vi "Add_Target.vi"(11 "Error_In":errorcluster) -> (4 "Target_Specification_Out":T1={"Target_Name"="LM233", "Register_Name"=["Register A", "Register B"], "Register_Address"=[0.0, 1.0], "Vmin"=0.0, "Vmax"=5.0, "Off_Set (uS)"=10.0, "T_HD_STA (uS)"=5.0, "T_HD_DAT (uS)"=5.0, "T_SU_DAT (uS)"=0.25, "Frequency (kHz)"=100.0, "T_SU_STO"=4.0, "T_Off (uS)"=5.0, "T_On (uS)"=5.0, "T_BUF"=5.0, "Sample_Per_Us"=1000.0, "Target_Type"=0, "Target_Address"=21} {"Target_Address" format="%x"; "Target_Type" items=["10 Bit Address", "7 Bit Address"]}, 15 "Error_Out":errorcluster)   [LabVIEW 2023]
uses:
  Controls/Add_Target_Specification_.ctl
  Controls/Menu_Ring.ctl
  Controls/Button.ctl
  Controls/Queue_Operation.ctl
  Controls/State_and_Data.ctl
  Drivers/Queue_Driver/QD_Main.vi
panel:
  in  "Add":T3
  in  "Target_Specification_In":T1 {"Target_Address" format="%x"; "Target_Type" items=["10 Bit Address", "7 Bit Address"]}
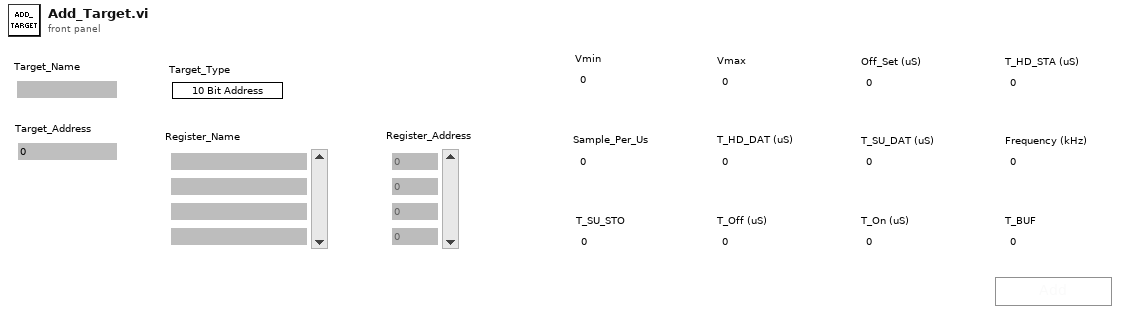
[diagram p1: front panel]
types:
  T1 = typedef "Add_Target_Specification_.ctl" = cluster{"Target_Name":string, "Register_Name":string[], "Register_Address":dbl[], "Vmin":dbl, "Vmax":dbl, "Off_Set (uS)":dbl, "T_HD_STA (uS)":dbl, "T_HD_DAT (uS)":dbl, "T_SU_DAT (uS)":dbl, "Frequency (kHz)":dbl, "T_SU_STO":dbl, "T_Off (uS)":dbl, "T_On (uS)":dbl, "T_BUF":dbl, "Sample_Per_Us":dbl, "Target_Type":T2, "Target_Address":u16}
  T2 = typedef "Menu_Ring.ctl" = u16
  T3 = typedef "Button.ctl" = bool
  T4 = typedef "Queue_Operation.ctl" = enum16{"Obtain_Queue", "Enqueue", "Enqueue_First", "Enqueue_N", "Lossy_Enqueue", "Preview", "Queue_Status", "Dequeue", "Flush", "Release_Queue"}
  T5 = typedef "State_and_Data.ctl" = cluster{"State":string, "Data":variant}
  T6 = enum32{"Invalid", "Standard", "Closed", "Hidden", "Minimized", "Maximized"}
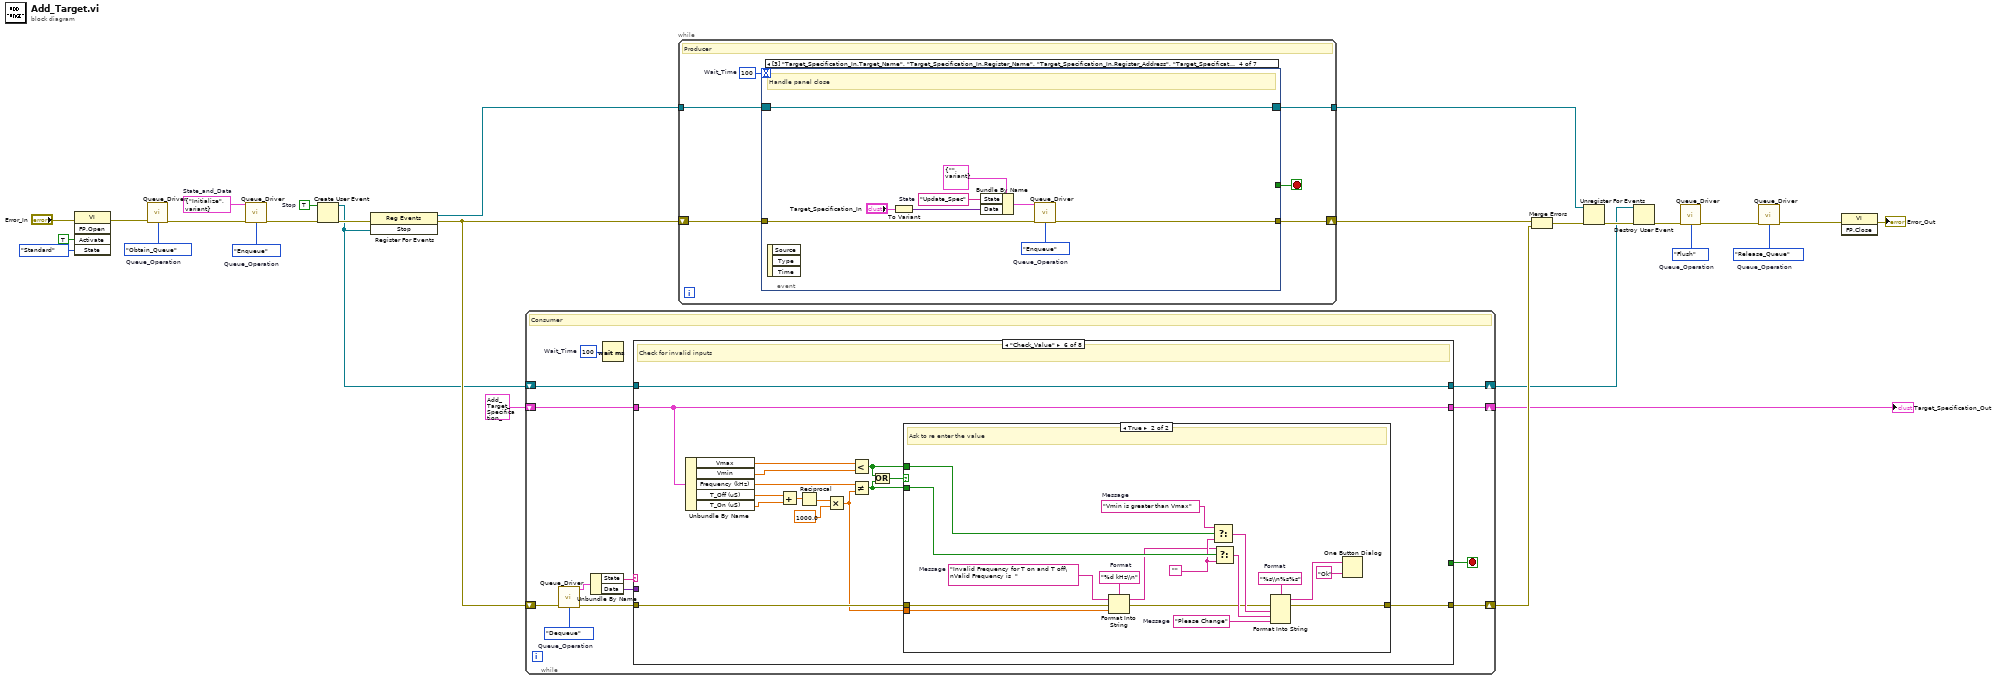
[diagram p0: block diagram]
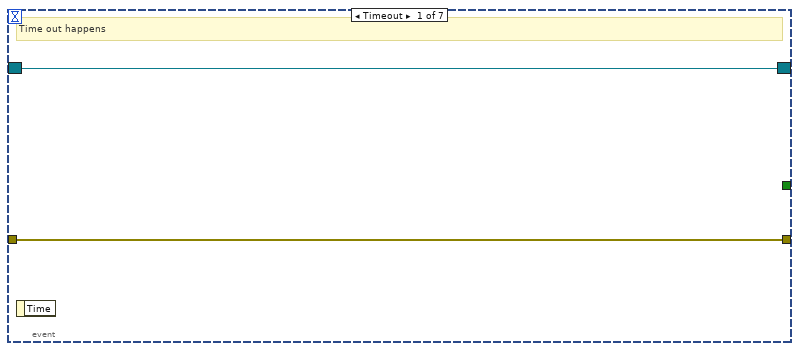
[diagram p2: hidden frame]
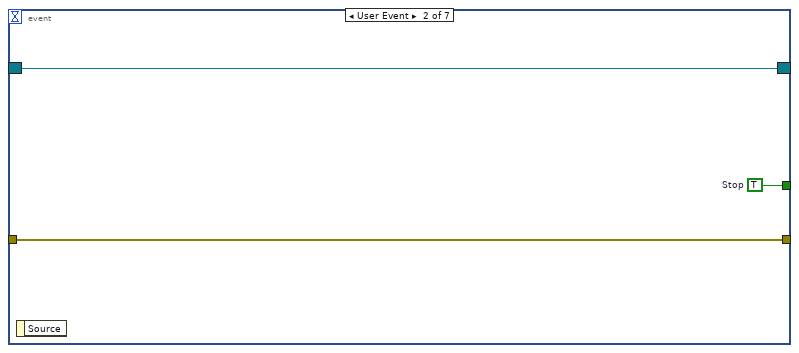
[diagram p3: hidden frame]
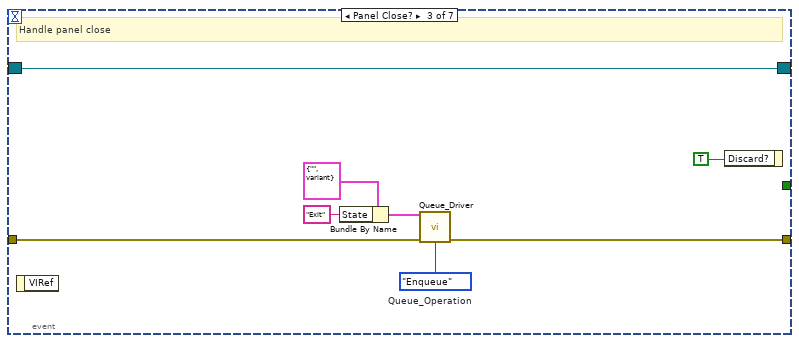
[diagram p4: hidden frame]
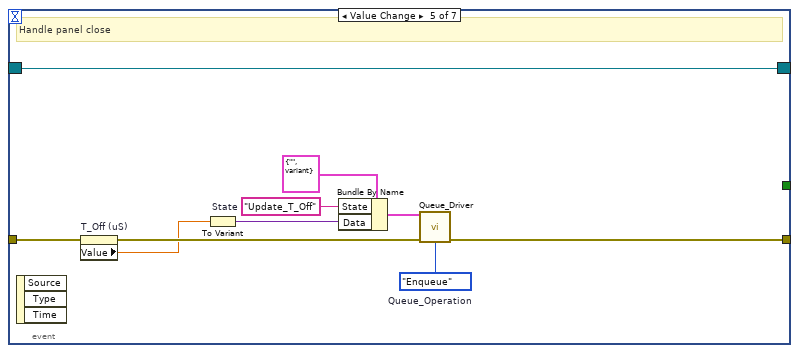
[diagram p5: hidden frame]
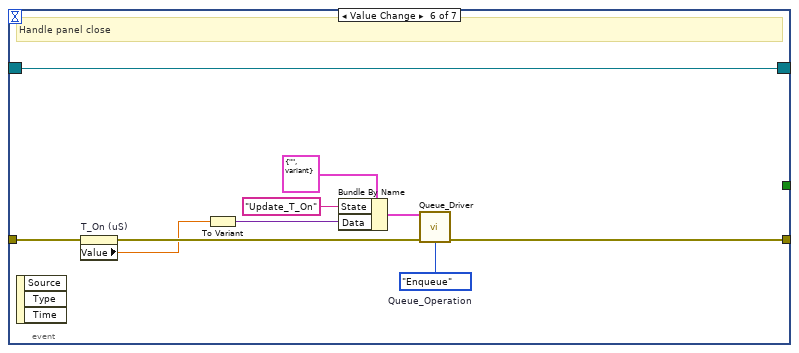
[diagram p6: hidden frame]
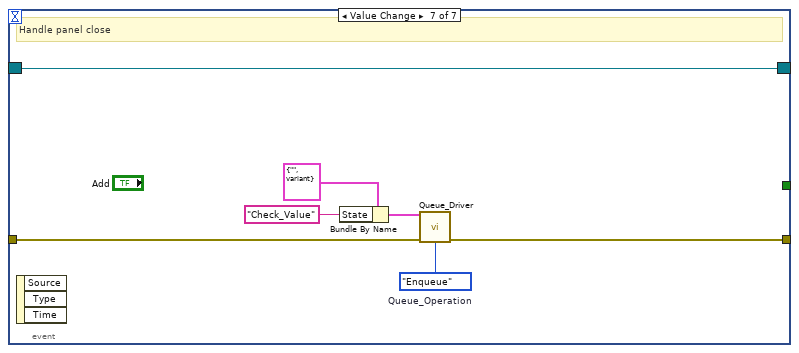
[diagram p7: hidden frame]
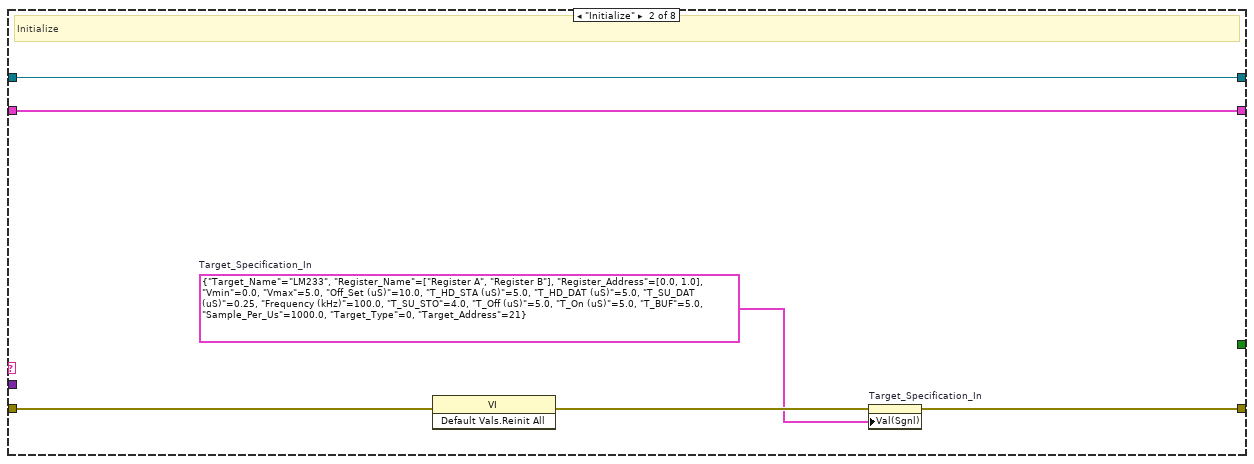
[diagram p9: hidden frame]
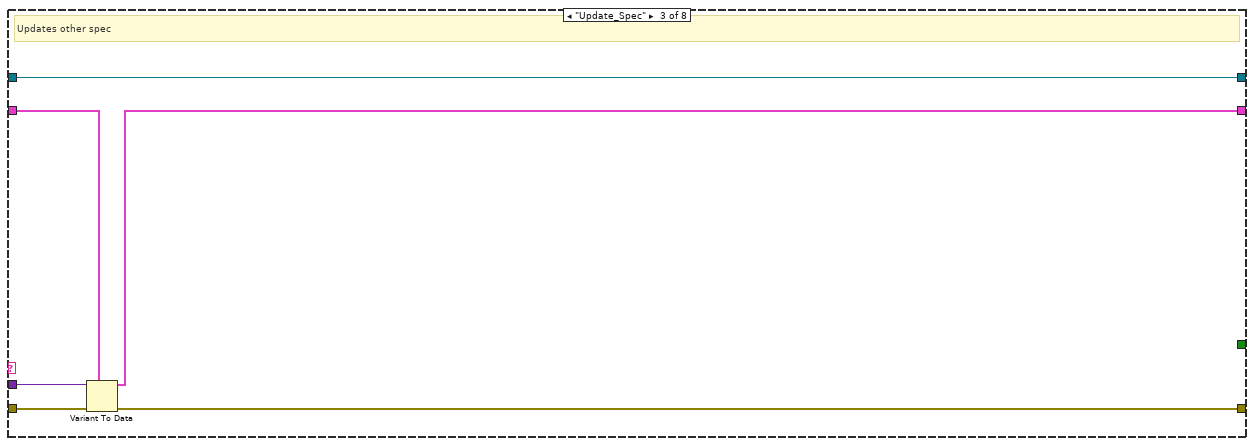
[diagram p10: hidden frame]
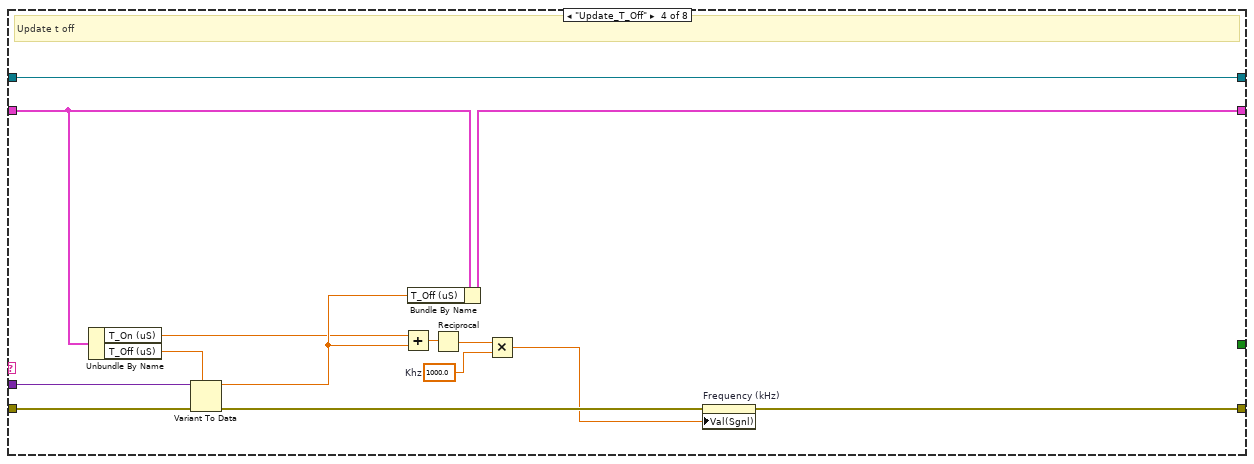
[diagram p11: hidden frame]
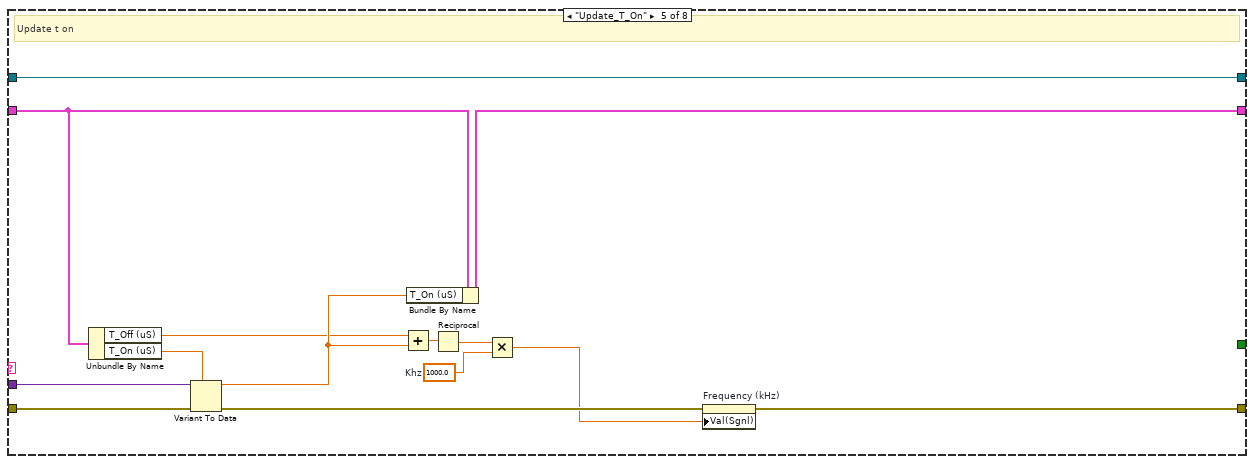
[diagram p12: hidden frame]
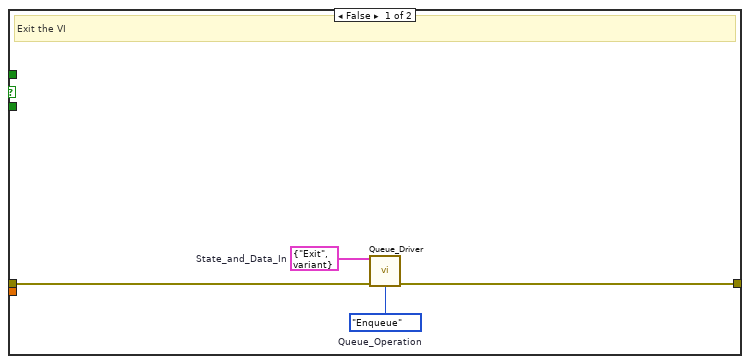
[diagram p13: hidden frame]
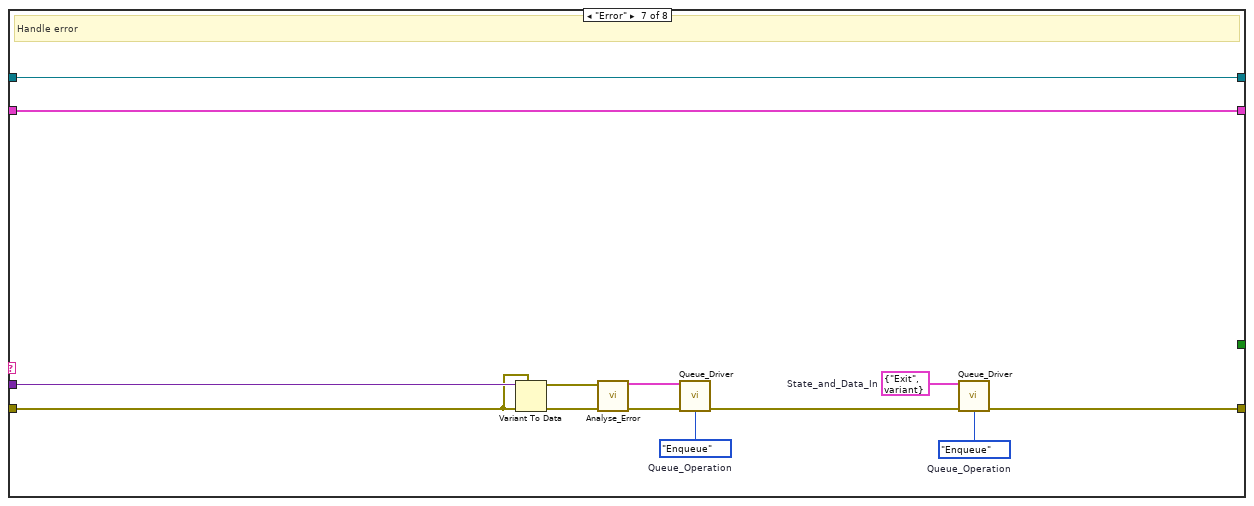
[diagram p14: hidden frame]
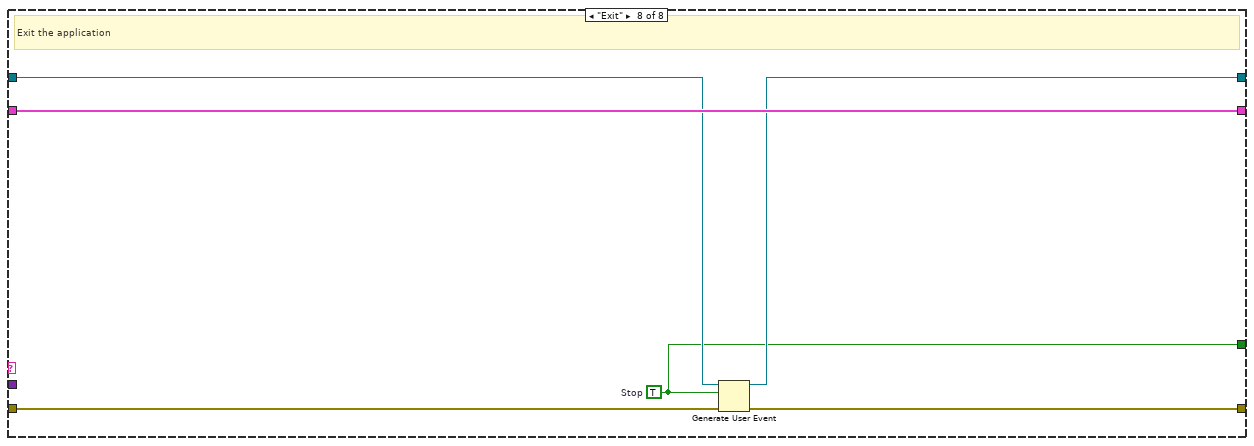
[diagram p15: hidden frame]
diagram:
  w8 = Queue_Operation."Release_Queue"  # Queue_Operation
  w9 = Queue_Operation."Flush"  # Queue_Operation
  w19 = TRUE  # Stop
  w21 = T5 {"State"="Initialize", "Data"=variant}  # State_and_Data
  w22 = Queue_Operation."Enqueue"  # Queue_Operation
  w23 = Queue_Operation."Obtain_Queue"  # Queue_Operation
  n1 = invoke class="VI" method="FP.Open"(error in="Error_In", "Activate"=TRUE ("Activate?"), "State"=T6."Standard") -> (error out=w4:errorcluster)  [unwired: 2 in, 4 out]
  n2 = call-poly "Queue_Driver.vi"("Error_In"=w4, "Queue_Operation"=w23) -> ("Error_Out"=w24:errorcluster)  [unwired: 11 in, 2 out]
  n3 = call-poly "Queue_Driver.vi"("State_and_Data_In"=w21, "Error_In"=w24, "Queue_Operation"=w22) -> ("Error_Out"=w7:errorcluster)  [unwired: 10 in, 2 out]
  n4 = Create User Event(user event datatype=w19, error in=w7) -> (user event=w5:refnum<user-event>, error out=w20:errorcluster)
  n5 = register-events(error in=w20, w5) -> (reference out=w18:refnum<event-registration>, error out=w6:errorcluster)  [unwired: 1 in]
  n6 = while {
    shift-right: [w33] -> w12
    shift-left: w5 -> [w34]
    shift-right: [w32] -> w1
    shift-left: T1 {"Target_Name"="LM233", "Register_Name"=["Register A", "Register B"], "Register_Address"=[0.0, 1.0], "Vmin"=0.0, "Vmax"=5.0, "Off_Set (uS)"=10.0, "T_HD_STA (uS)"=5.0, "T_HD_DAT (uS)"=5.0, "T_SU_DAT (uS)"=0.25, "Frequency (kHz)"=100.0, "T_SU_STO"=4.0, "T_Off (uS)"=5.0, "T_On (uS)"=5.0, "T_BUF"=5.0, "Sample_Per_Us"=1000.0, "Target_Type"=0, "Target_Address"=21} ("Target_Specification_In") -> [w35]
    shift-right: [w31] -> w16
    shift-left: w6 -> [w41]
    stop <- w30 stop-if-true
    w29 = u32 100  # Wait_Time
    w39 = Queue_Operation."Dequeue"  # Queue_Operation
    # "Consumer"
    n7 = call-poly "Queue_Driver.vi"("Error_In"=w41, "Queue_Operation"=w39) -> ("State_and_Data_Out"=w38:T5, "Error_Out"=w40:errorcluster)  [unwired: 11 in, 1 out]
    n8 = Unbundle By Name(w38) -> ("State"=w37:string, "Data"=w36:variant)
    n9 = Wait (ms)(milliseconds to wait=w29) -> ()  [unwired: 1 out]
    n10 = case shown="\"Check_Value\"" w37 {
      tunnel: [w44 w46 w54 w58 w72 w89 w124 w138] -> w31
      tunnel: w40 -> [w44 w49 w56 w70 w84 w100 w132 w140]
      tunnel: w36 -> [_ _ w53 w67 w81 _ w133 _]
      tunnel: w35 -> [w43 w48 w52 w66 w80 w98 w129 w139]
      tunnel: [w43 w48 w51 w64 w78 w98 w129 w139] -> w32
      tunnel: w34 -> [w42 w50 w55 w69 w83 w99 w134 w137]
      tunnel: [w42 w50 w55 w69 w83 w99 w134 w136] -> w33
      tunnel: [_ _ _ _ _ _ _ w135] -> w30
      frame Default {
      }
      frame "Initialize" {
        w45 = T1 {"Target_Name"="LM233", "Register_Name"=["Register A", "Register B"], "Register_Address"=[0.0, 1.0], "Vmin"=0.0, "Vmax"=5.0, "Off_Set (uS)"=10.0, "T_HD_STA (uS)"=5.0, "T_HD_DAT (uS)"=5.0, "T_SU_DAT (uS)"=0.25, "Frequency (kHz)"=100.0, "T_SU_STO"=4.0, "T_Off (uS)"=5.0, "T_On (uS)"=5.0, "T_BUF"=5.0, "Sample_Per_Us"=1000.0, "Target_Type"=0, "Target_Address"=21}  # Target_Specification_In
        # "Initialize"
        n11 = invoke class="VI" method="Default Vals.Reinit All"(error in=w49) -> (error out=w47:errorcluster)  [unwired: 2 in, 2 out]
        n12 = property on="Target_Specification_In" class="Clust (strict)"(error in=w47, "Val(Sgnl)"=w45) -> (error out=w46:errorcluster)  [unwired: 1 in, 1 out]
      }
      frame "Update_Spec" {
        # "Updates other spec"
        n13 = Variant To Data(error in=w56, type=w52, Variant=w53) -> (data=w51:T1, error out=w54:errorcluster)
      }
      frame "Update_T_Off" {
        w61 = 1000.0  # Khz
        # "Update t off"
        n14 = Unbundle By Name(w66) -> ("T_On (uS)"=w59:dbl, "T_Off (uS)"=w65:dbl)
        n15 = Variant To Data(error in=w70, type=w65, Variant=w67) -> (data=w60:dbl, error out=w68:errorcluster)
        n16 = Add(x=w59, y=w60) -> (x+y=w63:dbl)
        n17 = Bundle By Name(cluster=w66, "T_Off (uS)"=w60) -> (w64:T1)
        n18 = Reciprocal(x=w63) -> (1/x=w62:dbl)
        n19 = Multiply(x=w62, y=w61) -> (x*y=w57:dbl)
        n20 = property on="Frequency (kHz)" class="DigNum (strict)"(error in=w68, "Val(Sgnl)"=w57) -> (error out=w58:errorcluster)  [unwired: 1 in, 1 out]
      }
      frame "Update_T_On" {
        w75 = 1000.0  # Khz
        # "Update t on"
        n21 = Unbundle By Name(w80) -> ("T_Off (uS)"=w73:dbl, "T_On (uS)"=w79:dbl)
        n22 = Variant To Data(error in=w84, type=w79, Variant=w81) -> (data=w74:dbl, error out=w82:errorcluster)
        n23 = Add(x=w73, y=w74) -> (x+y=w77:dbl)
        n24 = Bundle By Name(cluster=w80, "T_On (uS)"=w74) -> (w78:T1)
        n25 = Reciprocal(x=w77) -> (1/x=w76:dbl)
        n26 = Multiply(x=w76, y=w75) -> (x*y=w71:dbl)
        n27 = property on="Frequency (kHz)" class="DigNum (strict)"(error in=w82, "Val(Sgnl)"=w71) -> (error out=w72:errorcluster)  [unwired: 1 in, 1 out]
      }
      frame "Check_Value" {
        # "Check for invalid inputs"
        n28 = Unbundle By Name(w98) -> ("Vmax"=w97:dbl, "Vmin"=w96:dbl, "Frequency (kHz)"=w90:dbl, "T_Off (uS)"=w95:dbl, "T_On (uS)"=w94:dbl)
        n29 = Add(x=w95, y=w94) -> (x+y=w93:dbl)
        n30 = Reciprocal(x=w93) -> (1/x=w92:dbl)
        n31 = Multiply(x=w92, y=1000.0) -> (x*y=w88:dbl)
        n32 = Less?(x=w97, y=w96) -> (x < y?=w86:bool)
        n33 = Not Equal?(x=w90, y=w88) -> (x != y?=w87:bool)
        n34 = Or(x=w86, y=w87) -> (x .or. y?=w85:bool)
        n35 = case shown="True" w85 {
          tunnel: w100 -> [w104 w121]
          tunnel: [w103 w120] -> w89
          tunnel: w86 -> [_ w117]
          tunnel: w87 -> [_ w114]
          tunnel: w88 -> [_ w108]
          frame False {
            w101 = T5 {"State"="Exit", "Data"=variant}  # State_and_Data_In
            w102 = Queue_Operation."Enqueue"  # Queue_Operation
            # "Exit the VI"
            n36 = call-poly "Queue_Driver.vi"("State_and_Data_In"=w101, "Error_In"=w104, "Queue_Operation"=w102) -> ("Error_Out"=w103:errorcluster)  [unwired: 10 in, 2 out]
          }
          frame True {
            w105 = "%s\\n%s%s"  # Format
            w106 = "%d kHz\\n"  # Format
            w111 = "Please Change"  # Message
            w112 = ""
            w109 = "Invalid Frequency for T on and T off\nValid Frequency is  "  # Message
            w116 = "Vmin is greater than Vmax"  # Message
            # "Ask to re enter the value"
            n37 = Format Into String(format string=w106, initial string=w109, error in=w121, w108) -> (resulting string=w107:string, error out=w110:errorcluster)
            n38 = Select(t=w116, s=w117, f=w112) -> (s? t:f=w115:string)
            n39 = Select(t=w107, s=w114, f=w112) -> (s? t:f=w113:string)
            n40 = Format Into String(format string=w105, error in=w110, w115, w113, w111) -> (resulting string=w119:string, error out=w120:errorcluster)  [unwired: 1 in]
            n41 = One Button Dialog(message=w119, button name ("OK")="Ok") -> ()  [unwired: 1 out]
          }
        }
      }
      frame "Error" {
        w122 = T5 {"State"="Exit", "Data"=variant}  # State_and_Data_In
        w123 = Queue_Operation."Enqueue"  # Queue_Operation
        w127 = Queue_Operation."Enqueue"  # Queue_Operation
        # "Handle error"
        n42 = Variant To Data(error in=w132, type=w132, Variant=w133) -> (data=w126:errorcluster, error out=w131:errorcluster)
        n43 = call "Analyse_Error.vi"("Erroe_Under_Analyse"=w126, "Error_In"=w131) -> ("State_and_Data"=w125:T5, "Error_Out"=w130:errorcluster)  [unwired: 12 in]
        n44 = call-poly "Queue_Driver.vi"("State_and_Data_In"=w125, "Error_In"=w130, "Queue_Operation"=w127) -> ("Error_Out"=w128:errorcluster)  [unwired: 10 in, 2 out]
        n45 = call-poly "Queue_Driver.vi"("State_and_Data_In"=w122, "Error_In"=w128, "Queue_Operation"=w123) -> ("Error_Out"=w124:errorcluster)  [unwired: 10 in, 2 out]
      }
      frame "Exit" {
        w135 = TRUE  # Stop
        # "Exit the application"
        n46 = Generate User Event(user event=w137, event data cluster=w135, error in=w140) -> (user event out=w136:refnum<user-event>, error out=w138:errorcluster)  [unwired: 1 in]
      }
    }
  }
  "Target_Specification_Out" <- w1
  n47 = while {
    tunnel: w18 -> [w145]
    shift-right: [w144] -> w17
    shift-left: w6 -> [w146]
    tunnel: [w142] -> w14
    stop <- w141 stop-if-true
    w143 = 100  # Wait_Time
    # "Producer"
    n48 = event shown="[3] \"Target_Specification_In.Target_Name\", \"Target_Specification_In.Register_Name\", \"Target_Specification_In.Register_Address\", \"Target_Specification_In.Vmin\", \"Target_Specification_In.Vmax\", \"Target_Specification_In.T_HD_STA (uS)\", \"Target_Specification_In.T_SU_DAT (uS)\", \"Target_Specification_In.Frequency (kHz)\", \"Target_Specification_In.T_SU_STO\", \"Target_Specification_In.T_BUF\", \"Target_Specification_In.Sample_Per_Us\", \"Target_Specification_In.Target_Type\", \"Target_Specification_In.Target_Address\": Value Change" {
      selector: w145 -> [w147 w149 w152 w163 w173 w183 w190]
      dyn-events: [w147 w149 w152 w163 w173 w183 w190] -> w142
      timeout: w143 -> [_ _ _ _ _ _ _]
      tunnel: w146 -> [w148 w150 w156 w167 w177 w187 w194]
      tunnel: [w148 w150 w155 w166 w176 w186 w193] -> w144
      tunnel: [_ w151 _ _ _ _ _] -> w141
      event Timeout {
        # "Time out happens"
        n49 = event-data() -> ()  [unwired: 1 in, 1 out]
      }
      event User Event {
        w151 = TRUE  # Stop
        n50 = event-data() -> ()  [unwired: 1 in, 1 out]
      }
      event Panel Close? {
        w157 = Queue_Operation."Enqueue"  # Queue_Operation
        # "Handle panel close"
        n51 = event-data() -> ()  [unwired: 1 in, 1 out]
        n52 = Bundle By Name(cluster=T5 {"State"="", "Data"=variant} ("State_and_Data"), "State"="Exit") -> (w154:T5)
        n53 = call-poly "Queue_Driver.vi"("State_and_Data_In"=w154, "Error_In"=w156, "Queue_Operation"=w157) -> ("Error_Out"=w155:errorcluster)  [unwired: 10 in, 2 out]
        n54 = event-data("Discard?"=TRUE) -> ()  [unwired: 1 in, 1 out]
      }
      event Value Change {
        w162 = "Update_Spec"  # State
        w168 = Queue_Operation."Enqueue"  # Queue_Operation
        # "Handle panel close"
        n55 = event-data() -> ()  [unwired: 1 in, 3 out]
        n56 = To Variant(anything="Target_Specification_In") -> (Variant=w160:variant)
        n57 = Bundle By Name(cluster=T5 {"State"="", "Data"=variant} ("State_and_Data"), "State"=w162, "Data"=w160) -> (w165:T5)
        n58 = call-poly "Queue_Driver.vi"("State_and_Data_In"=w165, "Error_In"=w167, "Queue_Operation"=w168) -> ("Error_Out"=w166:errorcluster)  [unwired: 10 in, 2 out]
      }
      event Value Change {
        w172 = "Update_T_Off"  # State
        w178 = Queue_Operation."Enqueue"  # Queue_Operation
        # "Handle panel close"
        n59 = event-data() -> ()  [unwired: 1 in, 3 out]
        n60 = property on="T_Off (uS)" class="DigNum (strict)"(error in=w177) -> (error out=w170:errorcluster, "Value"=w169:dbl)  [unwired: 1 in, 1 out]
        n61 = To Variant(anything=w169) -> (Variant=w171:variant)
        n62 = Bundle By Name(cluster=T5 {"State"="", "Data"=variant} ("State_and_Data"), "State"=w172, "Data"=w171) -> (w175:T5)
        n63 = call-poly "Queue_Driver.vi"("State_and_Data_In"=w175, "Error_In"=w170, "Queue_Operation"=w178) -> ("Error_Out"=w176:errorcluster)  [unwired: 10 in, 2 out]
      }
      event Value Change {
        w188 = Queue_Operation."Enqueue"  # Queue_Operation
        # "Handle panel close"
        n64 = event-data() -> ()  [unwired: 1 in, 3 out]
        n65 = property on="T_On (uS)" class="DigNum (strict)"(error in=w187) -> (error out=w180:errorcluster, "Value"=w179:dbl)  [unwired: 1 in, 1 out]
        n66 = To Variant(anything=w179) -> (Variant=w181:variant)
        n67 = Bundle By Name(cluster=T5 {"State"="", "Data"=variant} ("State_and_Data"), "State"="Update_T_On", "Data"=w181) -> (w185:T5)
        n68 = call-poly "Queue_Driver.vi"("State_and_Data_In"=w185, "Error_In"=w180, "Queue_Operation"=w188) -> ("Error_Out"=w186:errorcluster)  [unwired: 10 in, 2 out]
      }
      event Value Change {
        w195 = Queue_Operation."Enqueue"  # Queue_Operation
        # "Handle panel close"
        n69 = event-data() -> ()  [unwired: 1 in, 3 out]
        n70 = Bundle By Name(cluster=T5 {"State"="", "Data"=variant} ("State_and_Data"), "State"="Check_Value") -> (w192:T5)
        n71 = call-poly "Queue_Driver.vi"("State_and_Data_In"=w192, "Error_In"=w194, "Queue_Operation"=w195) -> ("Error_Out"=w193:errorcluster)  [unwired: 10 in, 2 out]
      }
    }
  }
  n72 = Merge Errors(w17, w16) -> (w15:errorcluster)
  n73 = Unregister For Events(event registration refnum=w14, error in=w15) -> (error out=w13:errorcluster)
  n74 = Destroy User Event(user event=w12, error in=w13) -> (error out=w11:errorcluster)
  n75 = call-poly "Queue_Driver.vi"("Error_In"=w11, "Queue_Operation"=w9) -> ("Error_Out"=w10:errorcluster)  [unwired: 11 in, 2 out]
  n76 = call-poly "Queue_Driver.vi"("Error_In"=w10, "Queue_Operation"=w8) -> ("Error_Out"=w3:errorcluster)  [unwired: 11 in, 2 out]
  n77 = invoke class="VI" method="FP.Close"(error in=w3) -> (error out=→"Error_Out":errorcluster)  [unwired: 2 in, 2 out]
